vi "Load Define Value.vi"(8 "error in (no error)":errorcluster) -> (0 "error out":errorcluster)   [LabVIEW 2020, in "DefineValue.lvlib"]
doc: "从文件加载控件默认值并初始化控件值"
uses:
  DefineValue.lvlib
  <vilib>/Utility/VariantDataType/VariantType.lvlib
panel:
  in  "VI_Reference":refnum<vi>
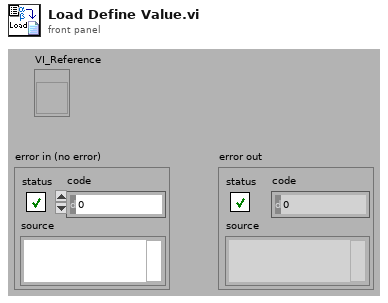
[diagram p1: front panel]
types:
  T1 = enum16{"open", "replace", "create", "open or create", "replace or create", "replace or create with confirmation"}
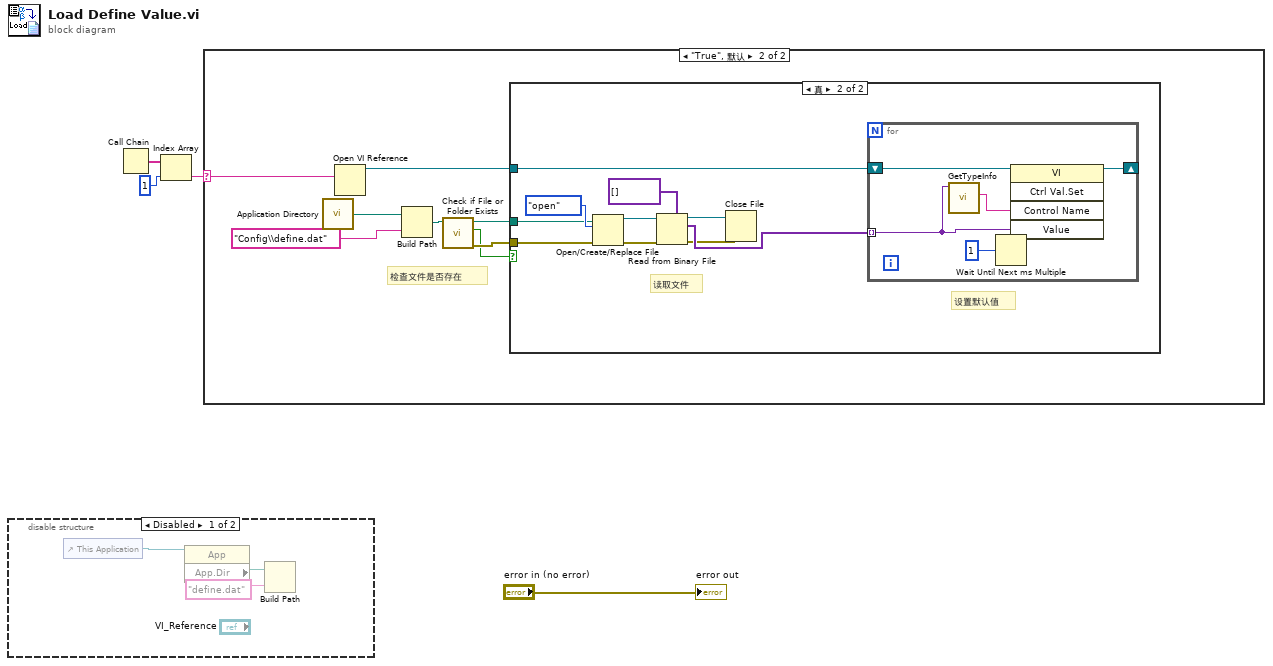
[diagram p0: block diagram]
diagram:
  n1 = disable-structure shown="Disabled" {
    frame Disabled {
      n2 = control-ref of="This Application"() -> (w7:refnum<vi>)
      n3 = property class="App"(reference=w7) -> ("App.Dir"=w5:path)  [unwired: 1 in, 2 out]
      n4 = Build Path(base path=w5, name or relative path="define.dat") -> ()  [unwired: 1 out]
    }
    frame Enabled {
    }
  }
  n5 = Call Chain() -> (call chain=w3:string[])
  n6 = Index Array(array=w3, index=1 ("Index")) -> (element=w1:string)
  n7 = case shown="\"True\", 默认" w1 {
    selector: w1 -> [_ w9]
    frame "" {
    }
    frame "True", Default {
      # "检查文件是否存在"
      n8 = call <vilib>:"Application Directory.vi"() -> ("Application Directory"=w12:path)
      n9 = Open VI Reference(vi path=w9) -> (vi reference=w8:refnum<vi>)  [unwired: 5 in, 1 out]
      n10 = Build Path(base path=w12, name or relative path="Config\\define.dat") -> (appended path=w10:path)
      n11 = call <vilib>:"Check if File or Folder Exists.vi"("path"=w10) -> ("error out"=w15:errorcluster, "file or folder exists?"=w13:bool, "dup path"=w14:path)  [unwired: 8 in]
      n12 = case shown="真" w13 {
        tunnel: w14 -> [_ w18]
        tunnel: w15 -> [_ w17]
        tunnel: w8 -> [_ w16]
        frame False {
        }
        frame True {
          # "设置默认值"
          # "读取文件"
          n13 = Open/Create/Replace File(file path (use dialog)=w18, error in=w17, operation (0:open)=T1."open" ("运行（0:打开）")) -> (refnum out=w20:refnum<file>, error out=w21:errorcluster)  [unwired: 3 in, 1 out]
          n14 = Read from Binary File(5:variant[] [] ("数组"), 8:w21, 11:w20) -> (0:w22:errorcluster, 2:w25:variant[], 3:w23:refnum<file>)  [unwired: 3 in, 1 out]
          n15 = Close File(refnum=w23, error in=w22) -> ()  [unwired: 2 out]
          n16 = for {
            shift-right: [w29] -> _
            shift-left: w16 -> [w30]
            tunnel: w25 -> [w28] mode=indexing
            n17 = call <vilib>:"GetTypeInfo.vi"("Variant"=w28) -> ("Name"=w27:string)  [unwired: 6 in, 4 out]
            n18 = Wait Until Next ms Multiple(millisecond multiple=u32 1 ("毫秒倍数")) -> ()  [unwired: 1 out]
            n19 = invoke class="VI" method="Ctrl Val.Set"(reference=w30, "Control Name"=w27, "Value"=w28) -> (reference out=w29:refnum<vi>)  [unwired: 2 in, 4 out]
          }
        }
      }
    }
  }
  "error out" <- "error in (no error)"
